vi "ExcelFile.vi"(0 "읽기 경로":path=path "C:/Users/bsyim/Documents/LabVIEW Data/Vi_Code/Excel_File/Sample3_Worksheets_2.xlsx", 5 "File Name":string, 7 "Data(in)":string[][](array[string]), 9 "Work Sheet":i32, 11 "error in (no error)":errorcluster caption="에러 입력(에러 없음)", 12 "Read/Wirte(거짓:읽기)":bool, 13 "File 열기(참)":bool, 14 "폴더 열기(거짓)":bool) -> (4 "3-D Data(All WorkSheet)":string[][][](array[string]), 6 "2-D Data(out)":string[][](array[string]), 8 "Current Work Sheet":string, 10 "Work Sheets":i32=1 min=0 step=1, 15 "error out":errorcluster caption="에러 출력")   [LabVIEW 2010]
uses:
  <vilib>/Utility/NIReport.llb/NI_report.lvclass
  <vilib>/addons/_office/excel.llb/Excel Get Data ([str]).vi
  <vilib>/addons/_office/excel.llb/Excel Easy Table (str).vi
  <vilib>/addons/_office/NI_ReportGenerationToolkit.lvlib
  <vilib>/Utility/NIReport.llb/Excel/NI_Excel.lvclass
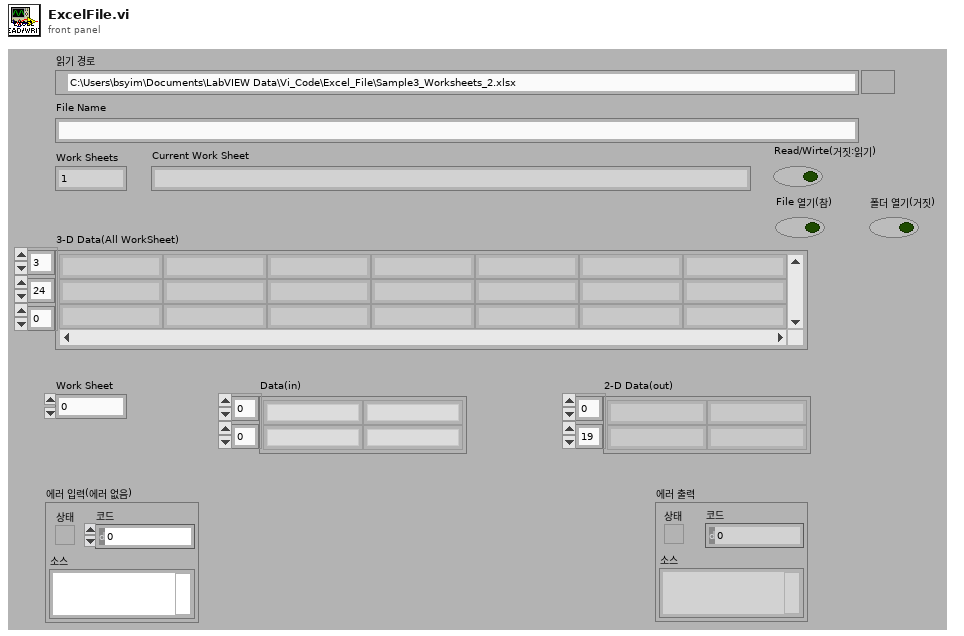
[diagram p1: front panel]
types:
  T1 = enum16{"Standard Report", "HTML", "Word", "Excel"}
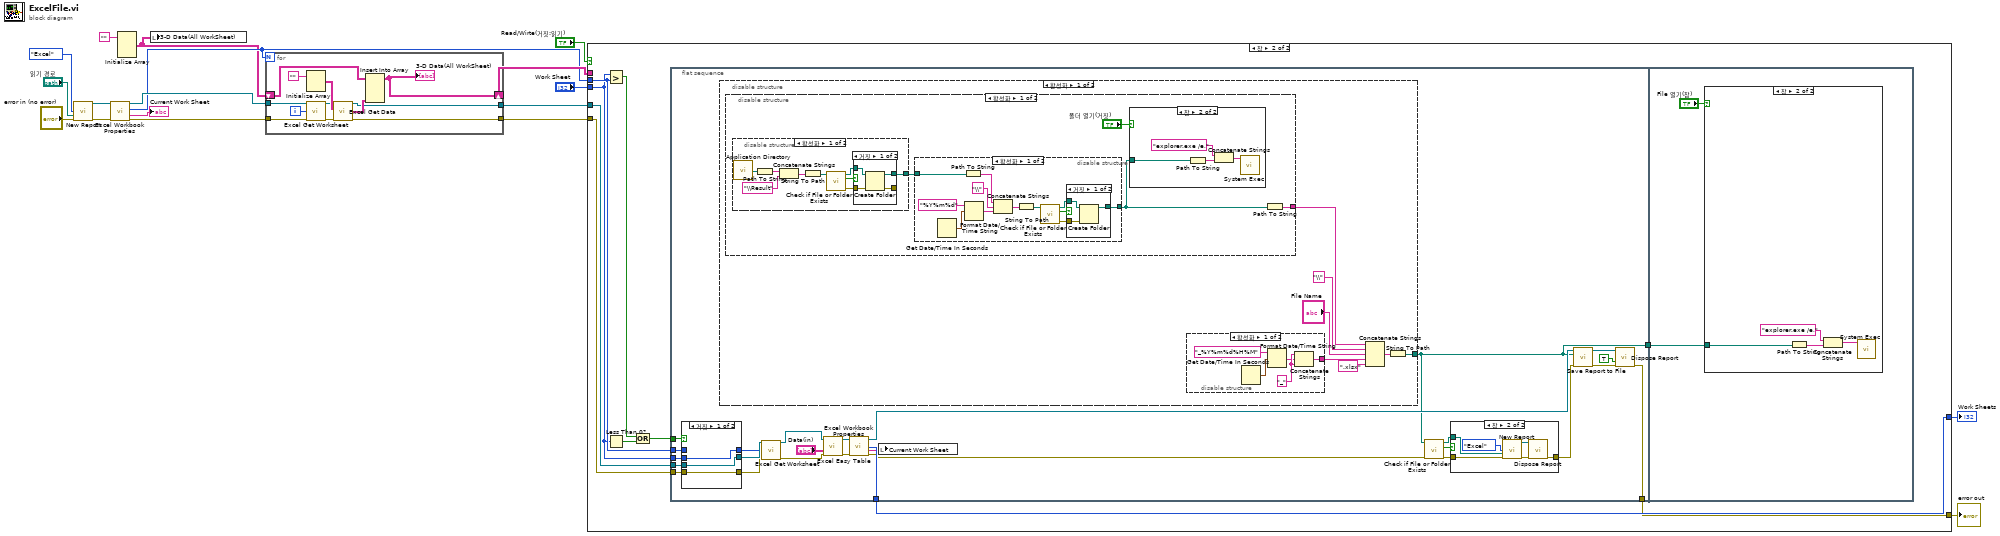
[diagram p0: block diagram]
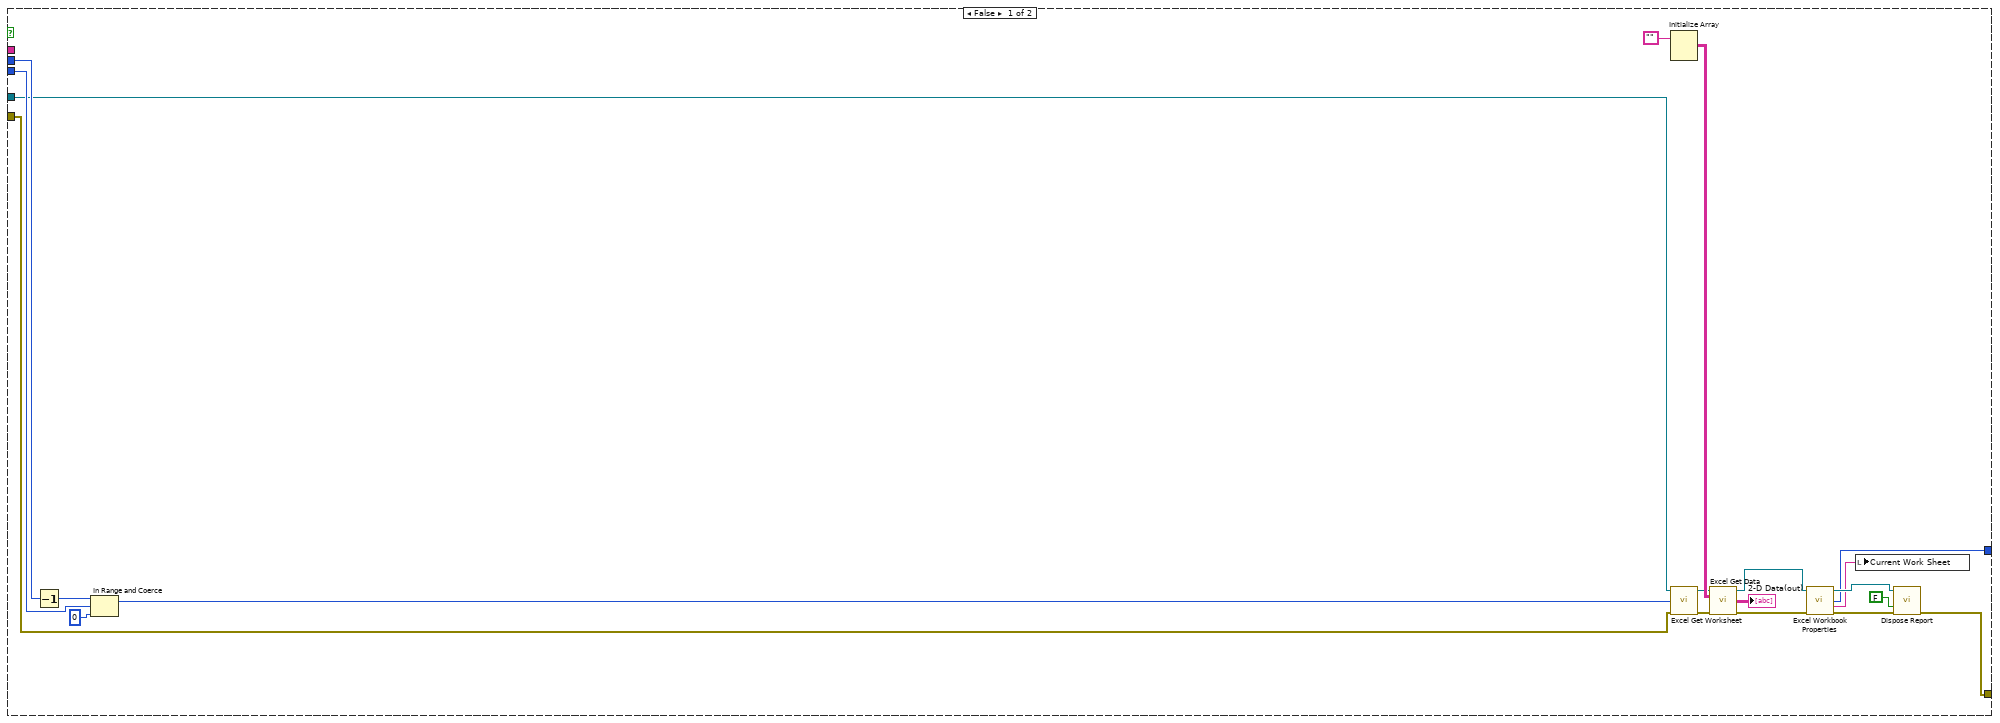
[diagram p2: hidden frame]
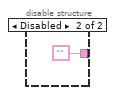
[diagram p10: hidden frame]
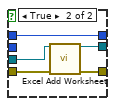
[diagram p12: hidden frame]
diagram:
  n1 = call <vilib>:"New Report.vi"("report type"=T1."Excel", "template (empty)"="읽기 경로", "error in (no error)"="error in (no error)") -> ("report out"=w12:refnum<class "NI_report.lvclass">, "error out"=w11:errorcluster)  [unwired: 11 in]
  n2 = call <vilib>:"Excel Workbook Properties.vi"("report in"=w12, "error in (no error)"=w11) -> ("report out"=w17:refnum<class "NI_report.lvclass">, "worksheets count"=w7:i32, "current worksheet name"=→"Current Work Sheet":string, "error out"=w15:errorcluster)  [unwired: 10 in]
  n3 = Initialize Array("") -> (w3:string[][][])  [unwired: 3 in]
  n4 = local write "3-D Data(All WorkSheet)"(w3) -> ()
  n5 = for {
    N: w7 -> [_]
    tunnel: w17 -> [w26]
    shift-right: [w23] -> w9
    shift-left: w3 -> [w28]
    tunnel: [w24] -> w13
    tunnel: w15 -> [w21]
    tunnel: [w19] -> w10
    i -> [w22]
    n6 = Initialize Array("") -> (w29:string[][])  [unwired: 2 in]
    n7 = call <vilib>:"Excel Get Worksheet.vi"("report in"=w26, "worksheet index (0)"=w22, "error in (no error)"=w21) -> ("report out"=w25:refnum<class "NI_report.lvclass">, "error out"=w20:errorcluster)  [unwired: 11 in]
    n8 = call-poly <vilib>:"Excel Get Data.vi"("report in"=w25, "data type"=w29, "error in (no error)"=w20) -> ("report out"=w24:refnum<class "NI_report.lvclass">, "data"=w27:string[][], "error out"=w19:errorcluster)  [unwired: 10 in]
    n9 = Insert Into Array(array=w28, new element=w27) -> (w23:string[][][])  [unwired: 3 in]
    "3-D Data(All WorkSheet)" <- w23
  }
  n10 = case shown="참" "Read/Wirte(거짓:읽기)" {
    tunnel: [w46 w52] -> w5
    tunnel: w13 -> [w36 w54]
    tunnel: w10 -> [w34 w55]
    tunnel: w9 -> [_ _]
    tunnel: w7 -> [w50 w57]
    tunnel: "Work Sheet" -> [w49 w56]
    tunnel: [w42 w53] -> w4
    frame False {
      n11 = Decrement(x=w50) -> (x-1=w47:i32)
      n12 = In Range and Coerce(upper limit=w47, x=w49, lower limit=0) -> (coerced(x)=w33:i32)  [unwired: 1 out]
      n13 = Initialize Array("") -> (w40:string[][])  [unwired: 2 in]
      n14 = call <vilib>:"Excel Get Worksheet.vi"("report in"=w36, "worksheet index (0)"=w33, "error in (no error)"=w34) -> ("report out"=w39:refnum<class "NI_report.lvclass">, "error out"=w38:errorcluster)  [unwired: 11 in]
      n15 = call-poly <vilib>:"Excel Get Data.vi"("report in"=w39, "data type"=w40, "error in (no error)"=w38) -> ("report out"=w37:refnum<class "NI_report.lvclass">, "data"=→"2-D Data(out)":string[][], "error out"=w35:errorcluster)  [unwired: 10 in]
      n16 = call <vilib>:"Excel Workbook Properties.vi"("report in"=w37, "error in (no error)"=w35) -> ("report out"=w44:refnum<class "NI_report.lvclass">, "worksheets count"=w42:i32, "current worksheet name"=w31:string, "error out"=w43:errorcluster)  [unwired: 10 in]
      n17 = local write "Current Work Sheet"(w31) -> ()
      n18 = call-dynamic "Dispose Report.vi"("report in"=w44, "save changes? (F)"=FALSE, "error in (no error)"=w43) -> ("error out"=w46:errorcluster)  [unwired: 12 in]
    }
    frame True {
      n19 = Greater?(x=w56, y=w57) -> (0:w60:bool)
      n20 = Less Than 0?(x=w56) -> (x < 0?=w59:bool)
      n21 = Or(x=w60, y=w59) -> (x .or. y?=w58:bool)
      n22 = flat-sequence {
        tunnel: w58 -> [w80]
        tunnel: w57 -> [w79]
        tunnel: w56 -> [w78]
        tunnel: w55 -> [w77]
        tunnel: w54 -> [w76]
        tunnel: [w72] -> w53
        tunnel: [w68] -> w52
        tunnel: [w65] -> w51
        tunnel: w51 -> [w155]
        frame #0 {
          n23 = case shown="거짓" w80 {
            tunnel: [w148 w153] -> w83
            tunnel: [w147 w152] -> w82
            tunnel: w77 -> [w147 w151]
            tunnel: w76 -> [w148 w150]
            tunnel: [w146 w149] -> w81
            tunnel: w79 -> [_ w149]
            tunnel: w78 -> [w146 _]
            frame False {
            }
            frame True {
              n24 = call <vilib>:"Excel Add Worksheet.vi"("report in"=w150, "error in (no error)"=w151) -> ("report out"=w153:refnum<class "NI_report.lvclass">, "error out"=w152:errorcluster)  [unwired: 12 in]
            }
          }
          n25 = disable-structure shown="활성화" {
            disable-tunnel: [w94 _] -> w65
            frame Enabled {
              n26 = disable-structure shown="활성화" {
                disable-tunnel: [w104 _] -> w96
                frame Enabled {
                  n27 = disable-structure shown="활성화" {
                    disable-tunnel: [w125 _] -> w103
                    frame Enabled {
                      n28 = call <vilib>:"Application Directory.vi"() -> ("Application Directory"=w133:path)
                      n29 = Path To String(path=w133) -> (string=w127:string)
                      n30 = Concatenate Strings(w127, "\\Result") -> (w126:string)
                      n31 = String To Path(string=w126) -> (path=w131:path)
                      n32 = call <vilib>:"Check if File or Folder Exists.vi"("path"=w131) -> ("error out"=w128:errorcluster, "file or folder exists?"=w130:bool, "dup path"=w129:path)  [unwired: 8 in]
                      n33 = case shown="거짓" w130 {
                        tunnel: w129 -> [w137 w138]
                        tunnel: w128 -> [w136 w139]
                        tunnel: [w135 w139] -> _
                        tunnel: [w134 w138] -> w125
                        frame False {
                          n34 = Create Folder(path (use dialog)=w137, error in=w136) -> (created path=w134:path, error out=w135:errorcluster)  [unwired: 1 in, 1 out]
                        }
                        frame True {
                        }
                      }
                    }
                    frame Disabled {
                    }
                  }
                  n35 = disable-structure shown="활성화" {
                    disable-tunnel: w103 -> [w111 _]
                    disable-tunnel: [w109 _] -> w102
                    frame Enabled {
                      n36 = Get Date/Time In Seconds() -> (seconds since 1Jan1904=w119:timestamp)
                      n37 = Path To String(path=w111) -> (string=w110:string)
                      n38 = Format Date/Time String(time format string (%c)="%Y%m%d", seconds (now)=w119) -> (date/time string=w118:string)  [unwired: 1 in]
                      n39 = Concatenate Strings(w110, "\\", w118) -> (w112:string)
                      n40 = String To Path(string=w112) -> (path=w113:path)
                      n41 = call <vilib>:"Check if File or Folder Exists.vi"("path"=w113) -> ("error out"=w114:errorcluster, "file or folder exists?"=w116:bool, "dup path"=w115:path)  [unwired: 8 in]
                      n42 = case shown="거짓" w116 {
                        tunnel: w115 -> [w123 w124]
                        tunnel: w114 -> [w122 _]
                        tunnel: [w121 w124] -> w109
                        frame False {
                          n43 = Create Folder(path (use dialog)=w123, error in=w122) -> (created path=w121:path)  [unwired: 1 in, 2 out]
                        }
                        frame True {
                        }
                      }
                    }
                    frame Disabled {
                    }
                  }
                  n44 = case shown="참" "폴더 열기(거짓)" {
                    tunnel: w102 -> [_ w108]
                    frame False {
                    }
                    frame True {
                      n45 = Path To String(path=w108) -> (string=w107:string)
                      n46 = Concatenate Strings("explorer.exe /e,", w107) -> (w105:string)
                      n47 = call <vilib>:"System Exec.vi"("command line"=w105) -> ()  [unwired: 7 in, 4 out]
                    }
                  }
                  n48 = Path To String(path=w102) -> (string=w104:string)
                }
                frame Disabled {
                }
              }
              n49 = disable-structure shown="활성화" {
                disable-tunnel: [w143 ""] -> w98
                frame Enabled {
                  w144 = "_"
                  n50 = Get Date/Time In Seconds() -> (seconds since 1Jan1904=w142:timestamp)
                  n51 = Format Date/Time String(time format string (%c)="_%Y%m%d%H%M", seconds (now)=w142) -> (date/time string=w141:string)  [unwired: 1 in]
                  n52 = Concatenate Strings(w144, w141, w144) -> (w143:string)
                }
                frame Disabled {
                }
              }
              n53 = Concatenate Strings(w96, "\\", "File Name", w98, ".xlsx") -> (w97:string)
              n54 = String To Path(string=w97) -> (path=w94:path)
            }
            frame Disabled {
            }
          }
          n55 = call <vilib>:"Excel Get Worksheet.vi"("report in"=w83, "worksheet index (0)"=w81, "error in (no error)"=w82) -> ("report out"=w85:refnum<class "NI_report.lvclass">, "error out"=w86:errorcluster)  [unwired: 11 in]
          n56 = call-poly <vilib>:"Excel Easy Table.vi"("report in"=w85, "text data"="Data(in)", "error in (no error)"=w86) -> ("report out"=w74:refnum<class "NI_report.lvclass">, "error out"=w73:errorcluster)  [unwired: 8 in, 3 out]
          n57 = call <vilib>:"Excel Workbook Properties.vi"("report in"=w74, "error in (no error)"=w73) -> ("report out"=w71:refnum<class "NI_report.lvclass">, "worksheets count"=w72:i32, "current worksheet name"=w61:string, "error out"=w67:errorcluster)  [unwired: 10 in]
          n58 = local write "Current Work Sheet"(w61) -> ()
          n59 = call <vilib>:"Check if File or Folder Exists.vi"("error in (no error)"=w67, "path"=w65) -> ("error out"=w62:errorcluster, "file or folder exists?"=w64:bool, "dup path"=w63:path)  [unwired: 7 in]
          n60 = case shown="참" w64 {
            tunnel: w63 -> [_ w92]
            tunnel: [w87 w91] -> w66
            tunnel: w62 -> [w87 w90]
            frame False {
            }
            frame True {
              n61 = call <vilib>:"New Report.vi"("report type"=T1."Excel", "template (empty)"=w92, "error in (no error)"=w90) -> ("report out"=w93:refnum<class "NI_report.lvclass">, "error out"=w89:errorcluster)  [unwired: 11 in]
              n62 = call-dynamic "Dispose Report.vi"("report in"=w93, "error in (no error)"=w89) -> ("error out"=w91:errorcluster)  [unwired: 13 in]
            }
          }
          n63 = call-dynamic "Save Report to File.vi"("report in"=w71, "report file path"=w65, "error in (no error)"=w66) -> ("report out"=w69:refnum<class "NI_report.lvclass">, "error out"=w70:errorcluster)  [unwired: 11 in]
          n64 = call-dynamic "Dispose Report.vi"("report in"=w69, "save changes? (F)"=TRUE, "error in (no error)"=w70) -> ("error out"=w68:errorcluster)  [unwired: 12 in]
        }
        frame #1 {
          n65 = case shown="참" "File 열기(참)" {
            tunnel: w155 -> [_ w159]
            frame False {
            }
            frame True {
              n66 = Path To String(path=w159) -> (string=w158:string)
              n67 = Concatenate Strings("explorer.exe /e,", w158) -> (w156:string)
              n68 = call <vilib>:"System Exec.vi"("command line"=w156) -> ()  [unwired: 7 in, 4 out]
            }
          }
        }
      }
    }
  }
  "error out" <- w5
  "Work Sheets" <- w4
